vi "Get_Driver_Commands.vi"() -> (3 "Driver Command_Inputs":T1)   [LabVIEW 2012]
uses:
  Command_Inputs.ctl
  tankdrive/Input_Commands_Drive.ctl
  Conveyor/Input_Command_Conveyor.ctl
  Turret/Inputs_Commands_Turret.ctl
  Bridge Tipper/Inputs_Tipper.ctl
  Dashboard Controls.ctl
  Roller/Input_Commands_Roller.ctl
  Flywheel/Input_Commands_Flywheel.ctl
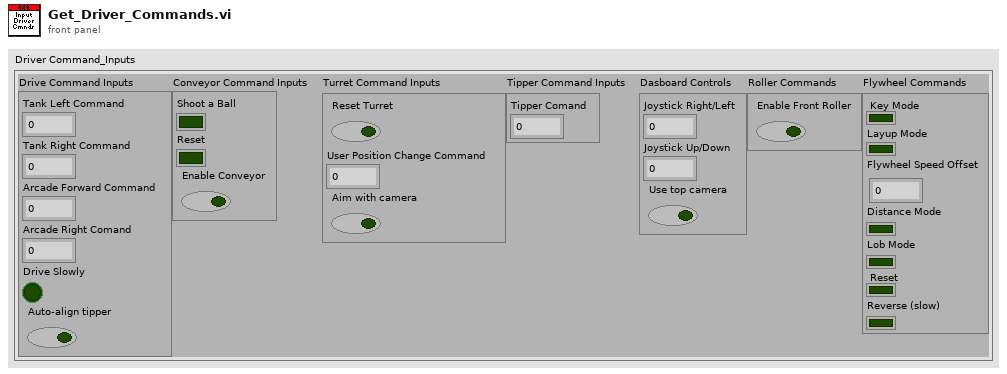
[diagram p1: front panel]
types:
  T1 = typedef "Command_Inputs.ctl" = cluster{"Drive Command Inputs":T2, "Conveyor Command Inputs":T3, "Turret Command Inputs":T4, "Tipper Command Inputs":T5, "Dasboard Controls":T6, "Roller Commands":T7, "Flywheel Commands":T8}
  T2 = typedef "Input_Commands_Drive.ctl" = cluster{"Tank Left Command":dbl, "Tank Right Command":dbl, "Arcade Forward Command":dbl, "Arcade Right Comand":dbl, "Drive Slowly":bool, "Auto-align tipper":bool}
  T3 = typedef "Input_Command_Conveyor.ctl" = cluster{"Shoot a Ball":bool, "Reset":bool, "Enable Conveyor":bool}
  T4 = typedef "Inputs_Commands_Turret.ctl" = cluster{"Reset Turret":bool, "User Position Change Command":dbl, "Aim with camera":bool}
  T5 = typedef "Inputs_Tipper.ctl" = cluster{"Tipper Comand":dbl}
  T6 = typedef "Dashboard Controls.ctl" = cluster{"Joystick Right/Left":dbl, "Joystick Up/Down":dbl, "Use top camera":bool}
  T7 = typedef "Input_Commands_Roller.ctl" = cluster{"Enable Front Roller":bool}
  T8 = typedef "Input_Commands_Flywheel.ctl" = cluster{"Key Mode":bool, "Layup Mode":bool, "Flywheel Speed Offset":dbl, "Distance Mode":bool, "Lob Mode":bool, "Reset":bool, "Reverse (slow)":bool}
  T9 = typedef "Input_All_Joysticks.ctl" = cluster{"Joystick 1":T10, "Joystick 2":T10, "Joystick 3":T10, "Joystick 4":T10}
  T10 = typedef "Input_Single_Joystick.ctl" = cluster{"Axes":cluster{"axis 1 (x)":dbl, "axis 2 (y)":dbl, "axis 3 (throttle)":dbl, "axis 4":dbl, "axis 5":dbl, "axis 6":dbl}, "Buttons":T11}
  T11 = typedef "WPI_JoystickButtonState.ctl" = cluster{"Button 1":bool, "Button 2":bool, "Button 3":bool, "Button 4":bool, "Button 5":bool, "Button 6":bool, "Button 7":bool, "Button 8":bool, "Button 9":bool, "Button 10":bool, "Button 11":bool, "Button 12":bool}
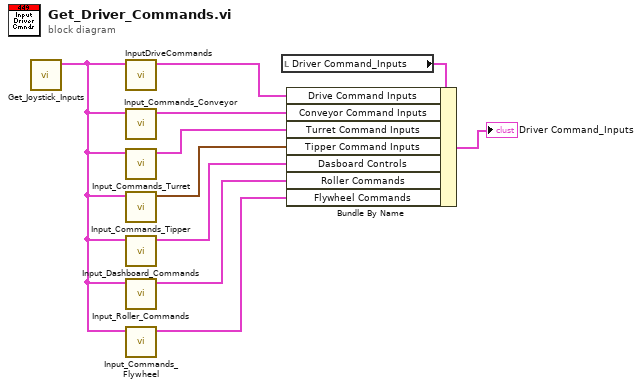
[diagram p0: block diagram]
diagram:
  n1 = call "Get_Joystick_Inputs.vi"() -> ("All Joysticks"=w1:T9)  [unwired: 11 in]
  n2 = call "InputDriveCommands.vi"("All Joysticks"=w1) -> ("Drive Command Inputs"=w8:T2)  [unwired: 10 in]
  n3 = call "Input_Commands_Conveyor.vi"("All Joysticks"=w1) -> ("Conveyor Command Inputs"=w7:T3)  [unwired: 10 in]
  n4 = call "Input_Commands_Turret.vi"("All Joysticks"=w1) -> ("Turret Command Inputs"=w6:T4)  [unwired: 10 in]
  n5 = call "Input_Commands_Tipper.vi"("All Joysticks"=w1) -> ("Tipper Command Inputs"=w5:T5)  [unwired: 10 in]
  n6 = call "Input_Dashboard_Commands.vi"("All Joysticks"=w1) -> ("Dashboard Controls"=w4:T6)  [unwired: 10 in]
  n7 = call "Input_Roller_Commands.vi"("All Joysticks"=w1) -> ("Roller Commands"=w3:T7)  [unwired: 10 in]
  n8 = call "Input_Commands_Flywheel.vi"("All Joysticks"=w1) -> ("Flywheel Commands"=w2:T8)  [unwired: 10 in]
  n9 = local read "Driver Command_Inputs"() -> (w10:T1)
  n10 = Bundle By Name(cluster=w10, "Drive Command Inputs"=w8, "Conveyor Command Inputs"=w7, "Turret Command Inputs"=w6, "Tipper Command Inputs"=w5, "Dasboard Controls"=w4, "Roller Commands"=w3, "Flywheel Commands"=w2) -> (→"Driver Command_Inputs":T1)
